vi "Auto Vision Main API.vi"(7 "Step No":i32, 8 "error in (no error)":errorcluster, 9 "SEQ Name":string, 11 "Data Cluster in":T1) -> (0 "error out":errorcluster, 3 "Data Cluster out":T1)   [LabVIEW 2020]
uses:
  controls/Auto UI Data.ctl
  controls/Configuration Details.ctl
  IPC/MQTT/Controls/Publish data.ctl
  IPC/MQTT/Q Driver/Controls/IPC-MQTT-Q driver-Q Options.ctl
  <vilib>/Utility/error.llb/whitespace.ctl
  <vilib>/vision/NI_Vision_Development_Module.lvlib
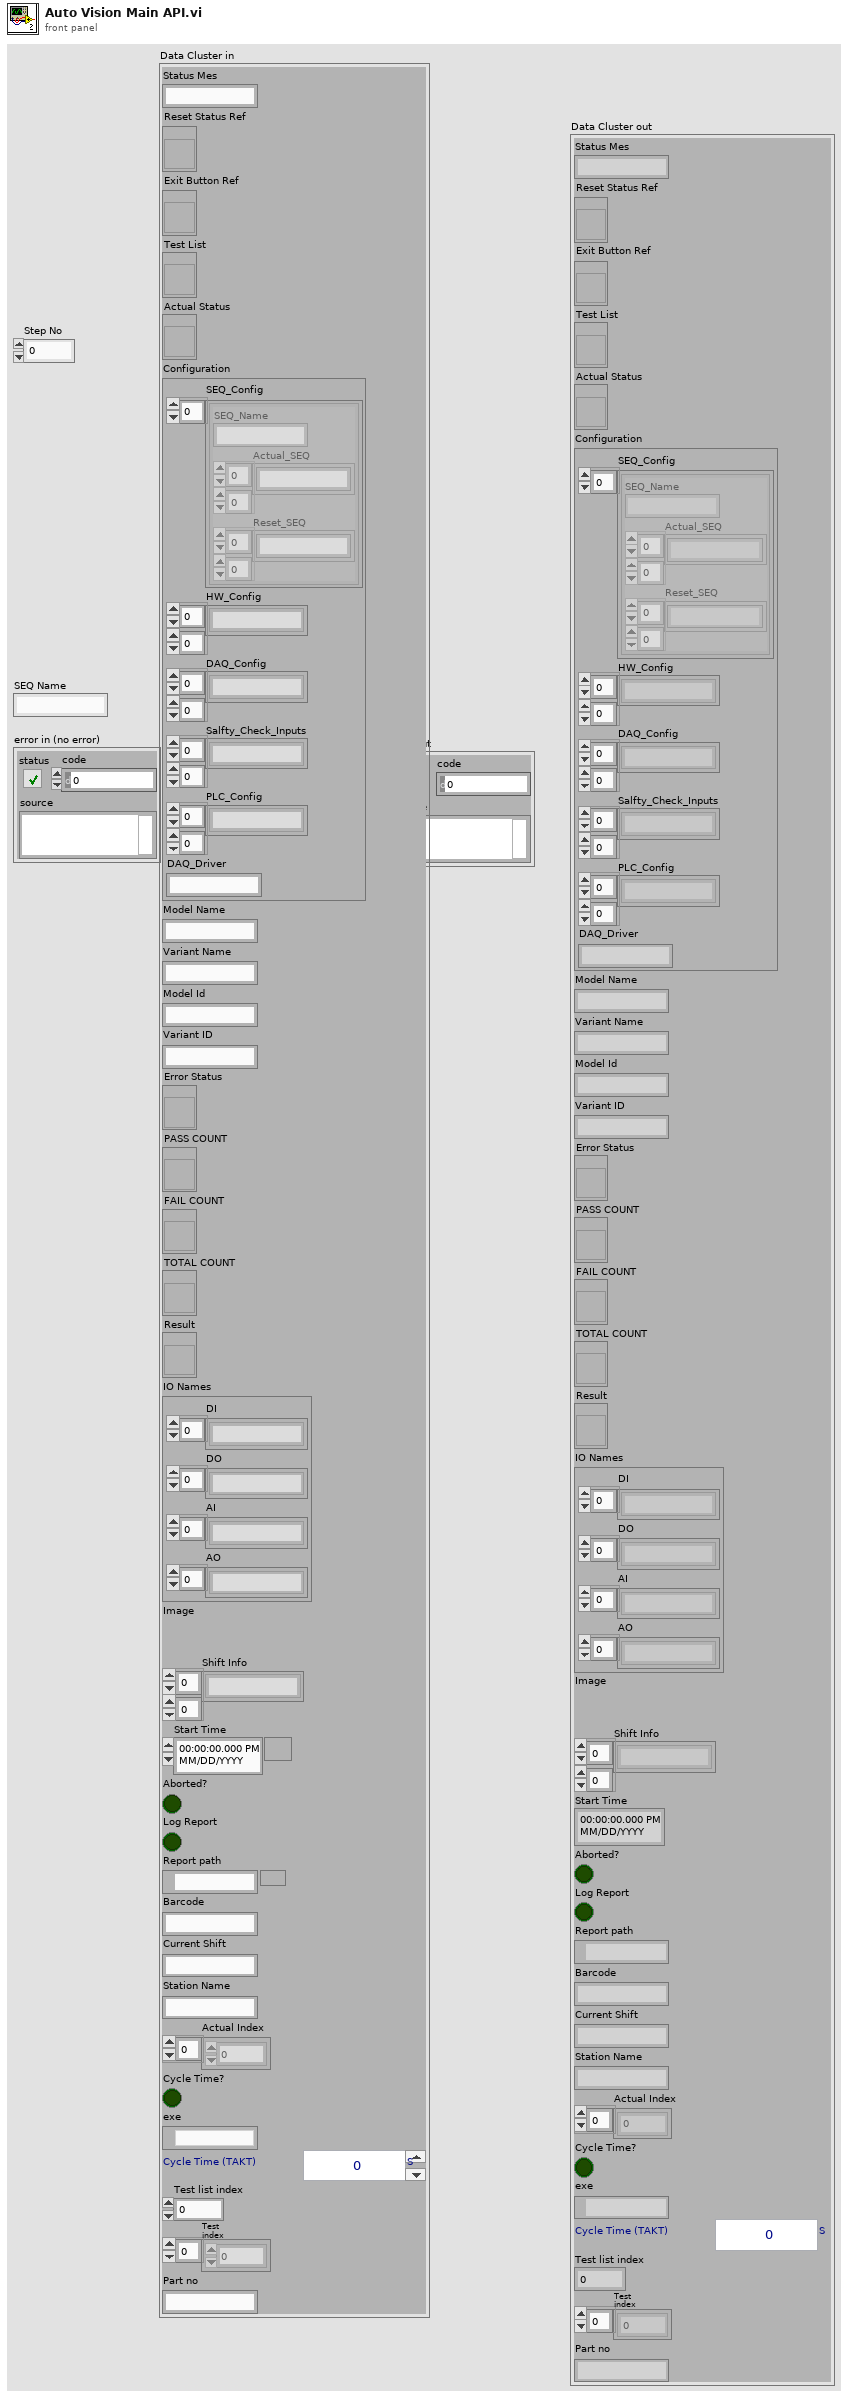
[diagram p1: front panel]
types:
  T1 = typedef "Auto UI Data.ctl" = cluster{"Status Mes":string, "Reset Status Ref":refnum<vi>, "Exit Button Ref":refnum<vi>, "Test List":refnum<vi>, "Actual Status":refnum<vi>, "Configuration":T2, "Model Name":string, "Variant Name":string, "Model Id":string, "Variant ID":string, "Error Status":refnum<vi>, "PASS COUNT":refnum<vi>, "FAIL COUNT":refnum<vi>, "TOTAL COUNT":refnum<vi>, "Result":refnum<vi>, "IO Names":cluster{"DI":string[], "DO":string[], "AI":string[], "AO":string[]}, "Image":T3, "Shift Info":string[][], "Start Time":timestamp, "Aborted?":bool, "Log Report":bool, "Report path":path, "Barcode":string, "Current Shift":string, "Station Name":string, "Actual Index":i32[], "Cycle Time?":bool, "exe":path, "Cycle Time (TAKT)":u16, "Test list index":u32, "Test index":u32[], "Part no":string}
  T2 = typedef "Configuration Details.ctl" = cluster{"SEQ_Config":cluster{"SEQ_Name":string, "Actual_SEQ":string[][], "Reset_SEQ":string[][]}[], "HW_Config":string[][], "DAQ_Config":string[][], "Salfty_Check_Inputs":string[][], "PLC_Config":string[][], "DAQ_Driver":string}
  T3 = typedef "IMAQ Image.ctl" = refnum<image>
  T4 = typedef "whitespace.ctl" = u16
  T5 = typedef "IPC-MQTT-Q driver-Q Options.ctl" = enum16{"En Q", "En Q N", "De Q", "Init", "En Q N Stack", "Flush", "Close"}
  T6 = typedef "Publish data.ctl" = cluster{"Topic":string, "Message":string}
  T7 = cluster{"SEQ_Name":string, "Actual_SEQ":string[][], "Reset_SEQ":string[][]}[]
  T8 = cluster{"Main_RGB":T3, "Temp_RGB":T3, "Main_Gray":T3, "Temp_Gray":T3}
  T9 = cluster{"Edge Score":dbl, "LL":dbl, "HL":dbl, " Result":bool}[]
  T10 = cluster{"Pattern Name":string, "Value":ext, "Area (pixels)":i32, "Result(Area pixels)":bool, "Pixel count Lower limit":i32, "Pixel count upper limit":i32, "Check Statistics":string, "Lower Limit":i32, "Upper Limit":i32, "Result":bool}[]
  T11 = cluster{"Pattern Name":string, "Pattern Score":dbl, "LL":dbl, "HL":dbl, "Pattern Result":bool}[]
  T12 = cluster{"Name":string, "Mini":dbl, "Max":dbl, "Value ":dbl, "Match":string, "Result":bool}[]
  T13 = cluster{"Name":string, "Mini":dbl, "Max":dbl, "Value ":dbl, "Result":bool}[]
  T14 = cluster{"Result":bool, "Exp value X":i64, "Exp value Y":i64, "Act value X ":i64, "Act value Y ":i64, "Name":string}
  T15 = cluster{"Name":string, "Mini":dbl, "Max":dbl, "Scaling ":dbl, "Value ":dbl, "Result":bool}[]
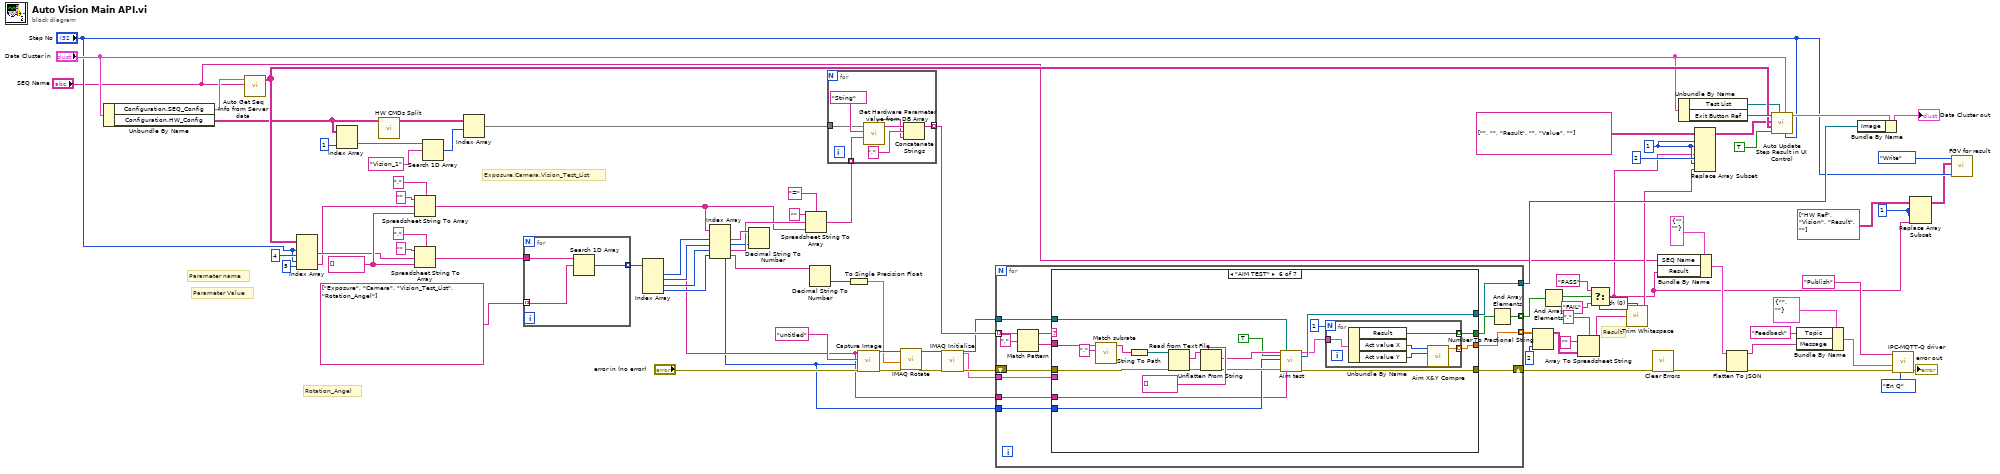
[diagram p0: block diagram]
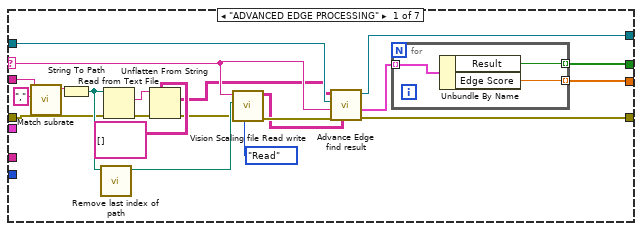
[diagram p2: hidden frame]
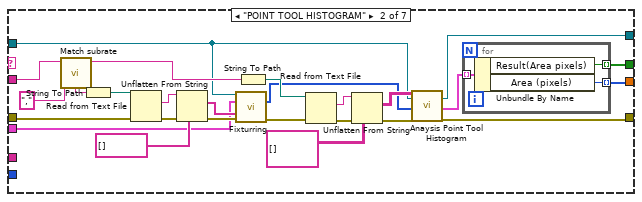
[diagram p3: hidden frame]
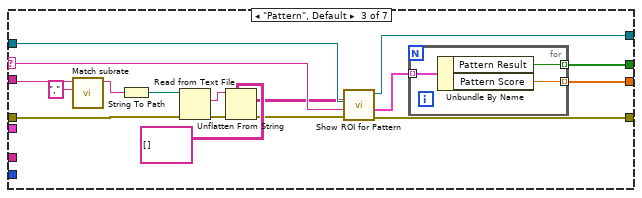
[diagram p4: hidden frame]
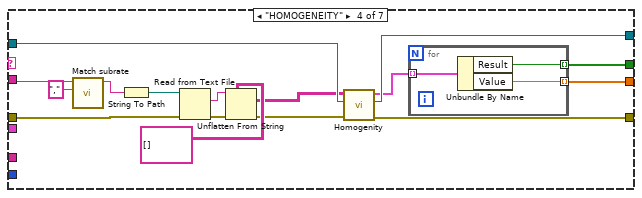
[diagram p5: hidden frame]
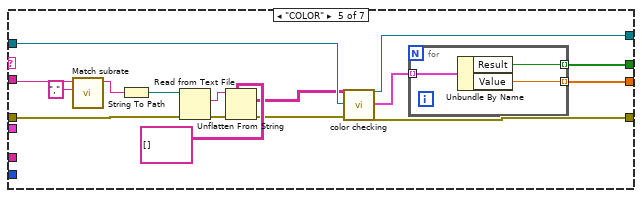
[diagram p6: hidden frame]
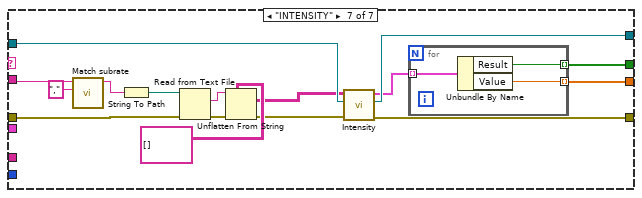
[diagram p7: hidden frame]
diagram:
  w1 = 1 ("index (row)")
  w23 = T4 0 items=["both", "start of string", "end of string"] ("location (both)")
  w38 = 1 ("index (row)")
  w70 = string[] []
  # "Rotation_Angel"
  # "Exposure,Camera,Vision_Test_List"
  # "Result"
  # "Parameter Value"
  # "Parameter name"
  n1 = Unbundle By Name("Data Cluster in") -> ("Configuration.SEQ_Config"=w32:T7, "Configuration.HW_Config"=w33:string[][])
  n2 = call "Auto Get Seq Info from Server data.vi"("SEQ Name"="SEQ Name", "SEQ_Config"=w32) -> ("Reset_SEQ"=w42:string[][])  [unwired: 8 in, 1 out]
  n3 = Index Array(array=w42, index (row) #1="Step No", index (col) #1=4 ("disabled index (col)"), index (row) #2="Step No", index (col) #2=5 ("disabled index (col)")) -> (element #1=w65:string, element #2=w64:string)
  n4 = Index Array(array=w33, index (col)=1 ("disabled index (col)")) -> (element=w77:string[])  [unwired: 1 in]
  n5 = call "HW CMDs Split.vi"("queryresult"=w33) -> ("Array"=w76:string[][])  [unwired: 10 in]
  n6 = Spreadsheet String To Array(delimiter (Tab)=",", format string="", spreadsheet string=w64, array type (2D Dbl)=w70) -> (array=w56:string[])
  n7 = Spreadsheet String To Array(delimiter (Tab)=",", format string="", spreadsheet string=w65, array type (2D Dbl)=w70) -> (array=w71:string[])
  n8 = Search 1D Array(1D array=w77, element="Vision_1") -> (index of element=w75:i32)  [unwired: 1 in]
  n9 = Index Array(array=w76, index (row)=w75) -> (element=w74:string[])  [unwired: 1 in]
  n10 = for {
    tunnel: w71 -> [w90]
    tunnel: string[] ["Exposure", "Camera", "Vision_Test_List", "Rotation_Angel"] -> [w89] mode=indexing
    tunnel: [w88] -> w63 mode=indexing
    n11 = Search 1D Array(1D array=w90, element=w89) -> (index of element=w88:i32)  [unwired: 1 in]
  }
  n12 = Index Array(array=w63) -> (element #1=w62:i32, element #2=w61:i32, element #3=w60:i32, element #4=w14:i32)  [unwired: 4 in]
  n13 = Index Array(array=w56, index #1=w62, index #2=w61, index #3=w60, index #4=w14) -> (element #1=w59:string, element #2=w10:string, element #3=w57:string, element #4=w15:string)
  n14 = Decimal String To Number(string=w59) -> (number=w9:i32)  [unwired: 2 in, 1 out]
  n15 = Spreadsheet String To Array(delimiter (Tab)="=", format string="", spreadsheet string=w57, array type (2D Dbl)=w56) -> (array=w53:string[])
  n16 = Decimal String To Number(string=w15) -> (number=w17:i32)  [unwired: 2 in, 1 out]
  n17 = for {
    tunnel: w74 -> [w96]
    tunnel: w53 -> [w95] mode=indexing
    tunnel: [w93] -> w31 mode=indexing
    n18 = call "Get Hardware Parameter value from DB Array.vi"("Parameter Name"=w95, "Data Type"="String", "Data"=w96) -> ("String"=w94:string, "Unit"=w91:string)  [unwired: 4 in, 3 out]
    n19 = Concatenate Strings(w94, "," ("string"), w91) -> (w93:string)
  }
  n20 = To Single Precision Float(number=w17) -> (single precision float=w16:sgl)
  n21 = call "Capture Image.vi"("error in (no error)"="error in (no error)", "Exposure"=w9, "String"="untitled", "Refnum in"=w10) -> ("error out"=w18:errorcluster, "Refnum out"=w20:T3)  [unwired: 6 in]
  n22 = call "IMAQ Rotate"("error in (no error)"=w18, "Angle (degrees)"=w16, "Image Src"=w20) -> ("error out"=w13:errorcluster, "Image Dst Out"=w19:T3)  [unwired: 7 in]
  n23 = call "IMAQ Initialize.vi"("error in"=w13) -> ("error out"=w12:errorcluster, "Multiple Image Cluster"=w11:T8)  [unwired: 9 in]
  n24 = for {
    tunnel: w19 -> [w108]
    tunnel: w31 -> [w107] mode=indexing
    shift-right: [w111] -> w73
    shift-left: w12 -> [w101]
    tunnel: [w106] -> w48 mode=indexing
    tunnel: [w103] -> w51 mode=indexing
    tunnel: [w105] -> w35
    tunnel: w11 -> [w100]
    tunnel: w10 -> [w99]
    tunnel: w9 -> [w98]
    n25 = Match Pattern(string=w107, regular expression=",") -> (before substring=w109:string, after substring=w102:string)  [unwired: 1 in, 2 out]
    n26 = case shown="\"AIM TEST\"" w109 {
      selector: w109 -> [w126 _ w179 _ _ _ _]
      tunnel: [w132 w161 w181 w200 w219 w242 w263] -> w111
      tunnel: w101 -> [w116 w149 w169 w189 w208 w232 w252]
      tunnel: w108 -> [w130 w140 w180 w199 w218 w241 w262]
      tunnel: [w131 w139 w178 w198 w217 w240 w261] -> w105
      tunnel: [w128 w137 w176 w196 w215 w238 w259] -> w104
      tunnel: [w127 w136 w175 w195 w214 w237 w258] -> w103
      tunnel: w102 -> [w114 w154 w167 w187 w206 w230 w250]
      tunnel: w100 -> [_ w141 _ _ _ _ _]
      tunnel: w99 -> [_ _ _ _ _ w224 _]
      tunnel: w98 -> [_ _ _ _ _ w225 _]
      frame "ADVANCED EDGE PROCESSING" {
        n27 = call "Match subrate.vi"("regular expression"=",", "data string 3"=w114) -> ("Before"=w112:string)  [unwired: 8 in, 1 out]
        n28 = String To Path(string=w112) -> (path=w118:path)
        n29 = call "Remove last index of path.vi"("Path"=w118) -> ("path"=w117:path)  [unwired: 10 in]
        n30 = Read from Text File(file (use dialog)=w118, error in=w116) -> (text=w122:string, error out=w121:errorcluster)  [unwired: 2 in, 2 out]
        n31 = Unflatten From String(type=string[][] [] ("Reset_SEQ"), binary string=w122, error in (no error)=w121) -> (value=w119:string[][], error out=w115:errorcluster)  [unwired: 2 in, 1 out]
        n32 = call "Vision Scaling file Read write.vi"("Enum"=enum16{"Write", "Read"}."Read", "error in (no error)"=w115, "dup path"=w117, "Vision tool"=w126) -> ("error out"=w124:errorcluster, "all rows"=w123:string[][])  [unwired: 6 in]
        n33 = call "Advance Edge find result.vi"("Scalling Value"=w123, "error in (no error)"=w124, "Vision Tool"=w126, "Image"=w130, "List box Value"=w119) -> ("error out"=w132:errorcluster, "ADVANCED EDGE PROCESSING Result"=w129:T9, "Image"=w131:T3)  [unwired: 4 in]
        n34 = for {
          tunnel: w129 -> [w135] mode=indexing
          tunnel: [w134] -> w128 mode=indexing
          tunnel: [w133] -> w127 mode=indexing
          n35 = Unbundle By Name(w135) -> ("Result"=w134:bool, "Edge Score"=w133:dbl)
        }
      }
      frame "POINT TOOL HISTOGRAM" {
        n36 = call "Match subrate.vi"("regular expression"=",", "data string 3"=w154) -> ("After"=w148:string, "Before"=w152:string)  [unwired: 8 in]
        n37 = String To Path(string=w148) -> (path=w147:path)
        n38 = Read from Text File(file (use dialog)=w147, error in=w149) -> (text=w150:string, error out=w151:errorcluster)  [unwired: 2 in, 2 out]
        n39 = Unflatten From String(type=string[] [] ("Reset_SEQ"), binary string=w150, error in (no error)=w151) -> (value=w143:string[], error out=w145:errorcluster)  [unwired: 2 in, 1 out]
        n40 = call "Fixturring.vi"("Image CRL"=w140, "Main In"=w141, "Referance Listbox"=w143, "error in"=w145) -> ("Fixturing ROI"=w142:i32[], "error out"=w144:errorcluster)  [unwired: 4 in, 6 out]
        n41 = String To Path(string=w152) -> (path=w160:path)
        n42 = Read from Text File(file (use dialog)=w160, error in=w144) -> (text=w159:string, error out=w158:errorcluster)  [unwired: 2 in, 2 out]
        n43 = Unflatten From String(type=string[][] [] ("Reset_SEQ"), binary string=w159, error in (no error)=w158) -> (value=w155:string[][], error out=w156:errorcluster)  [unwired: 2 in, 1 out]
        n44 = call "Anaysis Point Tool Histogram.vi"("Pointer Listbox Detail"=w155, "Image"=w140, "Fixturing ROI"=w142, "error in"=w156) -> ("Image"=w139:T3, "Array"=w138:T10, "error out"=w161:errorcluster)  [unwired: 12 in, 1 out]
        n45 = for {
          tunnel: w138 -> [w164] mode=indexing
          tunnel: [w163] -> w137 mode=indexing
          tunnel: [w162] -> w136 mode=indexing
          n46 = Unbundle By Name(w164) -> ("Result(Area pixels)"=w163:bool, "Area (pixels)"=w162:i32)
        }
      }
      frame "Pattern", Default {
        n47 = call "Match subrate.vi"("regular expression"=",", "data string 3"=w167) -> ("Before"=w165:string)  [unwired: 8 in, 1 out]
        n48 = String To Path(string=w165) -> (path=w174:path)
        n49 = Read from Text File(file (use dialog)=w174, error in=w169) -> (text=w173:string, error out=w172:errorcluster)  [unwired: 2 in, 2 out]
        n50 = Unflatten From String(type=string[][] [] ("Reset_SEQ"), binary string=w173, error in (no error)=w172) -> (value=w170:string[][], error out=w168:errorcluster)  [unwired: 2 in, 1 out]
        n51 = call "Show ROI for Pattern.vi"("error in (no error)"=w168, "Vision tool"=w179, "Image"=w180, "multi coloum list box"=w170) -> ("error out"=w181:errorcluster, "Pattern Rsult"=w177:T11, "Image 3"=w178:T3)  [unwired: 5 in]
        n52 = for {
          tunnel: w177 -> [w184] mode=indexing
          tunnel: [w183] -> w176 mode=indexing
          tunnel: [w182] -> w175 mode=indexing
          n53 = Unbundle By Name(w184) -> ("Pattern Result"=w183:bool, "Pattern Score"=w182:dbl)
        }
      }
      frame "HOMOGENEITY" {
        n54 = call "Match subrate.vi"("regular expression"=",", "data string 3"=w187) -> ("Before"=w185:string)  [unwired: 8 in, 1 out]
        n55 = String To Path(string=w185) -> (path=w194:path)
        n56 = Read from Text File(file (use dialog)=w194, error in=w189) -> (text=w193:string, error out=w192:errorcluster)  [unwired: 2 in, 2 out]
        n57 = Unflatten From String(type=string[][] [] ("Reset_SEQ"), binary string=w193, error in (no error)=w192) -> (value=w190:string[][], error out=w188:errorcluster)  [unwired: 2 in, 1 out]
        n58 = call "Homogenity.vi"("error in (no error)"=w188, "Image in"=w199, "Intensity Limit"=w190) -> ("error out"=w200:errorcluster, "Image out"=w198:T3, "Homogeneity"=w197:T12)  [unwired: 6 in]
        n59 = for {
          tunnel: w197 -> [w203] mode=indexing
          tunnel: [w202] -> w196 mode=indexing
          tunnel: [w201] -> w195 mode=indexing
          n60 = Unbundle By Name(w203) -> ("Result"=w202:bool, "Value"=w201:dbl)
        }
      }
      frame "COLOR" {
        n61 = call "Match subrate.vi"("regular expression"=",", "data string 3"=w206) -> ("Before"=w204:string)  [unwired: 8 in, 1 out]
        n62 = String To Path(string=w204) -> (path=w213:path)
        n63 = Read from Text File(file (use dialog)=w213, error in=w208) -> (text=w212:string, error out=w211:errorcluster)  [unwired: 2 in, 2 out]
        n64 = Unflatten From String(type=string[][] [] ("Reset_SEQ"), binary string=w212, error in (no error)=w211) -> (value=w209:string[][], error out=w207:errorcluster)  [unwired: 2 in, 1 out]
        n65 = call "color checking.vi"("Color list"=w209, "Image in"=w218, "error in"=w207) -> ("Image Out"=w217:T3, "Color Result"=w216:T13, "error out"=w219:errorcluster)  [unwired: 22 in]
        n66 = for {
          tunnel: w216 -> [w222] mode=indexing
          tunnel: [w221] -> w215 mode=indexing
          tunnel: [w220] -> w214 mode=indexing
          n67 = Unbundle By Name(w222) -> ("Result"=w221:bool, "Value"=w220:dbl)
        }
      }
      frame "AIM TEST" {
        n68 = call "Match subrate.vi"("regular expression"=",", "data string 3"=w230) -> ("Before"=w228:string)  [unwired: 8 in, 1 out]
        n69 = String To Path(string=w228) -> (path=w236:path)
        n70 = Read from Text File(file (use dialog)=w236, error in=w232) -> (text=w235:string, error out=w234:errorcluster)  [unwired: 2 in, 2 out]
        n71 = Unflatten From String(type=string[] [] ("Reset_SEQ"), binary string=w235, error in (no error)=w234) -> (value=w227:string[], error out=w231:errorcluster)  [unwired: 2 in, 1 out]
        n72 = call "Aim test.vi"("List box Aiming"=w227, "Check path or camera"=TRUE, "Exposure"=w225, "error in 3"=w231, "Image"=w241, "Camera Refnum in"=w224) -> ("Aiming Result"=w239:T14, "Image 2"=w240:T3, "error out 3"=w242:errorcluster)  [unwired: 10 in, 1 out]
        n73 = for {
          N: 1 -> [_]
          tunnel: w239 -> [w247]
          tunnel: [w246] -> w238 mode=indexing
          tunnel: [w245] -> w237 mode=indexing
          n74 = Unbundle By Name(w247) -> ("Result"=w246:bool, "Act value X"=w244:i64, "Act value Y"=w243:i64)
          n75 = call "Aim X&Y Compre.vi"("Y"=w243, "X"=w244) -> ("X&Y cordinate"=w245:dbl)  [unwired: 9 in]
        }
      }
      frame "INTENSITY" {
        n76 = call "Match subrate.vi"("regular expression"=",", "data string 3"=w250) -> ("Before"=w248:string)  [unwired: 8 in, 1 out]
        n77 = String To Path(string=w248) -> (path=w257:path)
        n78 = Read from Text File(file (use dialog)=w257, error in=w252) -> (text=w256:string, error out=w255:errorcluster)  [unwired: 2 in, 2 out]
        n79 = Unflatten From String(type=string[][] [] ("Reset_SEQ"), binary string=w256, error in (no error)=w255) -> (value=w253:string[][], error out=w251:errorcluster)  [unwired: 2 in, 1 out]
        n80 = call "Intensity.vi"("error in (no error)"=w251, "Image in"=w262, "Intensity Limit"=w253) -> ("error out"=w263:errorcluster, "Image out"=w261:T3, "Intensity"=w260:T15)  [unwired: 6 in]
        n81 = for {
          tunnel: w260 -> [w266] mode=indexing
          tunnel: [w265] -> w259 mode=indexing
          tunnel: [w264] -> w258 mode=indexing
          n82 = Unbundle By Name(w266) -> ("Result"=w265:bool, "Value"=w264:dbl)
        }
      }
    }
    n83 = And Array Elements(Boolean array=w104) -> (logical AND=w106:bool)
  }
  n84 = Number To Fractional String(number=w51, precision (6)=i16 2) -> (F-format string=w22:string[][])  [unwired: 2 in]
  n85 = And Array Elements(Boolean array=w48) -> (logical AND=w47:bool)
  n86 = Array To Spreadsheet String(delimiter (Tab)=",", array=w22, 3:"" ("format string")) -> (spreadsheet string=w37:string)
  n87 = Select(t="PASS" ("Message"), s=w47, f="FAIL" ("Message")) -> (s? t:f=w2:string)
  n88 = call <vilib>:"Trim Whitespace.vi"("string"=w37, "location (both)"=w23) -> ("trimmed string"=w24:string)
  n89 = call <vilib>:"Clear Errors.vi"("error in (no error)"=w73) -> ("error out"=w28:errorcluster)  [unwired: 5 in, 1 out]
  n90 = Bundle By Name(cluster=cluster{"SEQ Name":string, "Result":string} {"SEQ Name"="", "Result"=""} ("Client FB"), "SEQ Name"="SEQ Name", "Result"=w2) -> (w26:cluster{"SEQ Name":string, "Result":string})
  n91 = Unbundle By Name("Data Cluster in") -> ("Test List"=w40:refnum<vi>, "Exit Button Ref"=w44:refnum<vi>)
  n92 = Replace Array Subset(array=string[][] [["", ""], ["Result", ""], ["Value", ""]] ("Step Result"), new element #1=w2, index (row) #1=w38, index (col) #1=w38, new element #2=w24, index (row) #2=2 ("index (row)"), index (col) #2=w38) -> (w5:string[][])
  n93 = Flatten To JSON(anything=w26, error in (no error)=w28) -> (JSON string=w25:string, 11:w27:errorcluster)  [unwired: 1 in]
  n94 = call "Auto Update Step Result in UI Control.vi"("Step No"="Step No", "Data Cluster in"="Data Cluster in", "Test List"=w40, "Acutal(T)/Reset(F)?"=TRUE, "Reset_SEQ"=w42, "Step Result"=w5, "Boolean in"=w44) -> ("Data Cluster out"=w45:T1)  [unwired: 4 in]
  n95 = Bundle By Name(cluster=T6 {"Topic"="", "Message"=""} ("Cluster"), "Topic"="Feedback", "Message"=w25) -> (w80:T6)
  n96 = Bundle By Name(cluster=w45, "Image"=w35) -> (→"Data Cluster out":T1)
  n97 = call "IPC-MQTT-Q driver.vi"("Q Options"=IPC-MQTT-Q_driver-Q_Options."En Q", "error in (no error)"=w27, "Message Data"=w80, "Message"="Publish") -> ("error out"=→"error out":errorcluster)  [unwired: 5 in, 2 out]
  n98 = Replace Array Subset(array=string[][] [["HW Ref", "Vision"], ["Result", ""]] ("Step Result"), new element=w2, index (row)=w1, index (col)=w1) -> (w4:string[][])
  n99 = call "FGV for result.vi"("Seq id in"="Step No", "In Data"=w4, "Enum"=enum16{"Ini", "Write", "Read"}."Write") -> ()  [unwired: 7 in, 2 out]
